vi "for_v0_v7.vi"() -> ()   [LabVIEW 2010]
panel:
  out "Numarul de iteratii":dbl=60.0
  in  "Iesire":bool
  in  "Stop":bool=TRUE
  in  "Slide":u8(slide)=60 scale=0.0..255.0
  out "Numeric":dbl=34.0
  out "Array":bool[](array[boolean])=[FALSE, FALSE, TRUE, FALSE, FALSE, FALSE, TRUE, FALSE]
  # "Start"
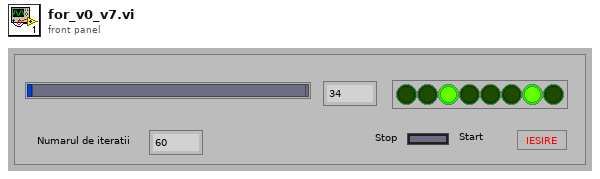
[diagram p1: front panel]
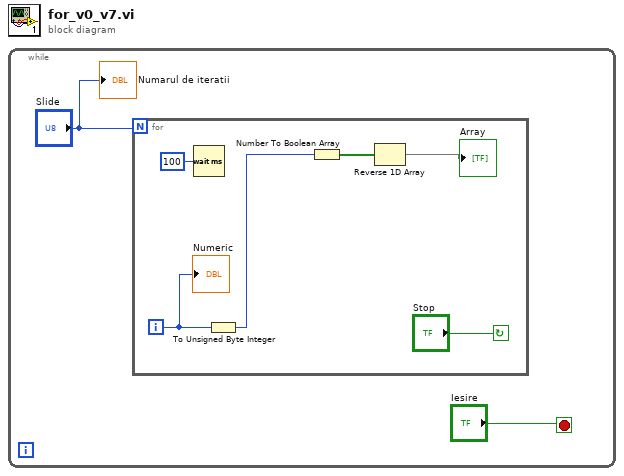
[diagram p0: block diagram]
diagram:
  n1 = while {
    stop <- "Iesire" stop-if-true
    n2 = for {
      N: "Slide" -> [_]
      i -> [w4]
      stop <- "Stop" continue-if-true
      n3 = Wait (ms)(milliseconds to wait=u32 100) -> ()  [unwired: 1 out]
      n4 = To Unsigned Byte Integer(number=w4) -> (unsigned 8bit integer=w5:u8)
      n5 = Number To Boolean Array(number=w5) -> (Boolean array=w8:bool[])
      n6 = Reverse 1D Array(array=w8) -> (reversed array=→"Array":bool[])
      "Numeric" <- w4
    }
    "Numarul de iteratii" <- "Slide"
  }
